vi "Set Top Level RD Data Path.vi"(8 "error in (no error)":errorcluster, 10 "Path":path, 11 "CRDS in":refnum<class "CRDS.lvclass">) -> (0 "error out":errorcluster, 3 "CRDS out":refnum<class "CRDS.lvclass">)   [LabVIEW 2014, in "CRDS.lvclass"]
uses:
  CRDS.lvclass
  File IO/Class/File Observer.lvclass
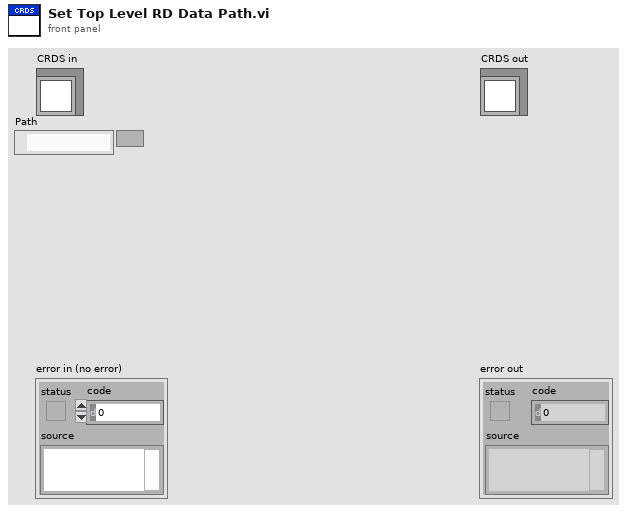
[diagram p1: front panel]
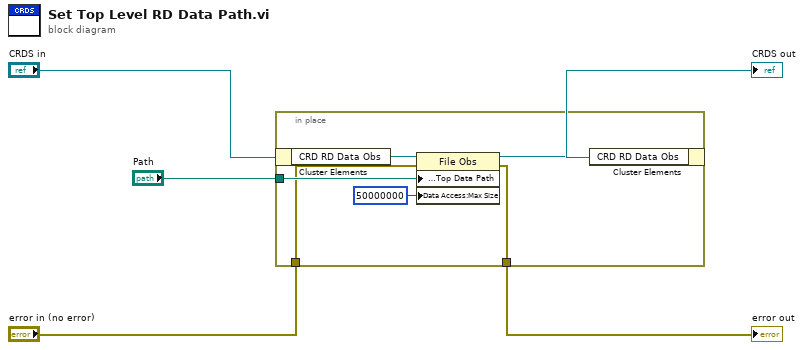
[diagram p0: block diagram]
diagram:
  n1 = in-place {
    in-place-border: "Path" -> [w10]
    in-place-border: "error in (no error)" -> [w7]
    in-place-border: [w6] -> w1
    n2 = in-place-cluster #1("CRDS in") -> ("CRD RD Data Obs"=w11:refnum<class "File Observer.lvclass">)
    n3 = property class="File Obs"(reference=w11, error in=w7, "Data Access:Top Data Path"=w10, "Data Access:Max Size"=i64 50000000 ("Max Size")) -> (reference out=w9:refnum<class "File Observer.lvclass">, error out=w6:errorcluster)
    n4 = in-place-cluster #1("CRD RD Data Obs"=w9) -> (→"CRDS out":refnum<class "CRDS.lvclass">)
  }
  "error out" <- w1
